vi "LEP_RV_LaunchCheckSpec.vi"(8 "error in (no error)":errorcluster) -> (0 "error out":errorcluster, 3 "OK":bool)   [LabVIEW 2011]
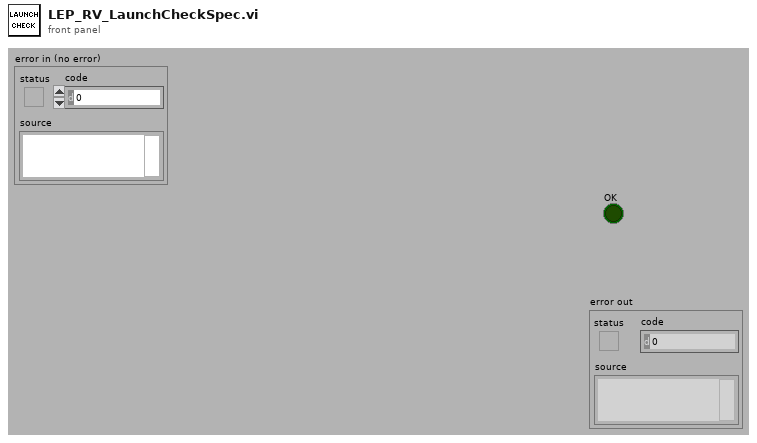
[diagram p1: front panel]
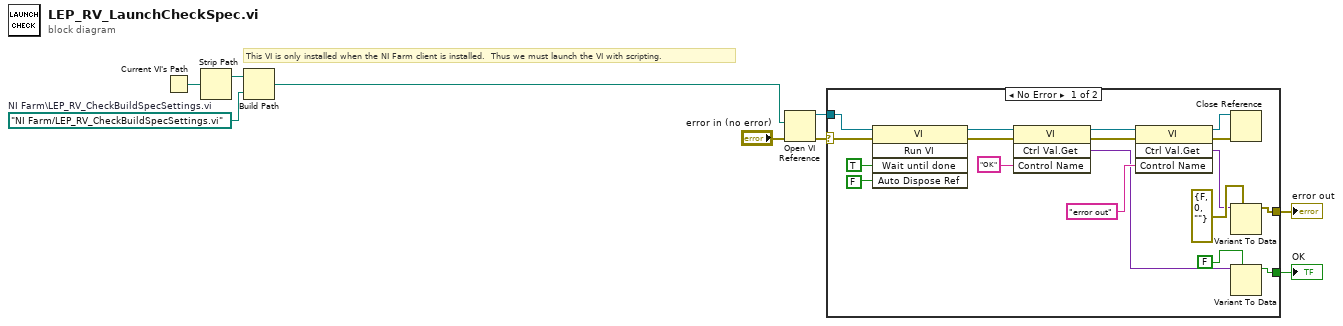
[diagram p0: block diagram]
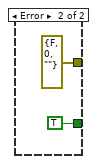
[diagram p2: hidden frame]
diagram:
  w9 = path "NI Farm/LEP_RV_CheckBuildSpecSettings.vi"  # NI Farm\LEP_RV_CheckBuildSpecSettings.vi
  # "This VI is only installed when the NI Farm client is installed.  Thus we must launch the VI with scripting."
  n1 = Current VI's Path() -> (path=w8:path)
  n2 = Strip Path(path=w8) -> (stripped path=w7:path)  [unwired: 1 out]
  n3 = Build Path(base path=w7, name or relative path=w9) -> (appended path=w6:path)
  n4 = Open VI Reference(vi path=w6, error in (no error)="error in (no error)") -> (vi reference=w5:refnum<vi>, error out=w4:errorcluster)  [unwired: 4 in]
  n5 = case shown="No Error" w4 {
    selector: w4 -> [w22 _]
    tunnel: w5 -> [w27 _]
    tunnel: [w17 TRUE ("OK")] -> w2
    tunnel: [w10 errorcluster {"status"=FALSE, "code"=0, "source"=""} ("error out")] -> w1
    frame No Error {
      n6 = invoke class="VI" method="Run VI"(reference=w27, error in=w22, "Wait until done"=TRUE ("Wait Until Done"), "Auto Dispose Ref"=FALSE ("Auto Dispose Reference")) -> (reference out=w24:refnum<vi>, error out=w23:errorcluster)  [unwired: 1 in, 3 out]
      n7 = invoke class="VI" method="Ctrl Val.Get"(reference=w24, error in=w23, "Control Name"="OK") -> (reference out=w21:refnum<vi>, error out=w20:errorcluster, "Get Control Value Variant"=w12:variant)  [unwired: 1 in, 1 out]
      n8 = invoke class="VI" method="Ctrl Val.Get"(reference=w21, error in=w20, "Control Name"="error out") -> (reference out=w16:refnum<vi>, error out=w15:errorcluster, "Get Control Value Variant"=w11:variant)  [unwired: 1 in, 1 out]
      n9 = Close Reference(reference=w16, error in (no error)=w15) -> ()  [unwired: 1 out]
      n10 = Variant To Data(type=errorcluster {"status"=FALSE, "code"=0, "source"=""} ("error out"), Variant=w11) -> (data=w10:errorcluster)  [unwired: 1 in, 1 out]
      n11 = Variant To Data(type=FALSE ("OK"), Variant=w12) -> (data=w17:bool)  [unwired: 1 in, 1 out]
    }
    frame Error {
    }
  }
  "OK" <- w2
  "error out" <- w1
